vi "抓圓.vi"(0 "Image In":T3, 1 "Process":T8(ring), 2 "Optimized Mode":bool, 3 "Direction":enum16{"Inner to Outer", "Outer to Inner"}(ring), 5 "ROI":T2, 7 "Coordinate System":T1 {"Measurement System"."Axis Reference" items=["Direct", "Indirect"]; "Measurement System"."Angle (deg)" format="%.2f"; "Measurement System"."Origin"."Y" format="%.2f"; "Measurement System"."Origin"."X" format="%.2f"; "Reference System"."Axis Reference" items=["Direct", "Indirect"]; "Reference System"."Angle (deg)" format="%.2f"; "Reference System"."Origin"."Y" format="%.2f"; "Reference System"."Origin"."X" format="%.2f"}, 9 "Gap":i32=10 min=1 max=300, 11 "error In":errorcluster, 12 "Edge Options":T6={"Edge Polarity"=0, "Kernel Size"=3, "Width"=3, "Minimum Edge Strength"=10.0, "Interpolation Type"=enum."Bilinear Fixed", "Data Processing Method"=enum."Average"} {"Edge Polarity" items=["All Edges", "Rising Edges", "Falling Edges"]; "Minimum Edge Strength" format="%.2f"; "Width" step=2; "Kernel Size" step=2}, 13 "Point Diameter (5)":u32=5 min=3 max=1000) -> (4 "Imag e Out":T3, 6 "Line Profile":T4(graph), 10 "Gradient Information":dbl[][](graph), 14 "Ellipse":T5 {"Minor Axis"."Point 2"."Y" format="%.2f"; "Minor Axis"."Point 2"."X" format="%.2f"; "Minor Axis"."Point 1"."Y" format="%.2f"; "Minor Axis"."Point 1"."X" format="%.2f"; "Major Axis"."Point 2"."Y" format="%.2f"; "Major Axis"."Point 2"."X" format="%.2f"; "Major Axis"."Point 1"."Y" format="%.2f"; "Major Axis"."Point 1"."X" format="%.2f"; "Center"."Y" format="%.2f"; "Center"."X" format="%.2f"}, 15 "error out":errorcluster)   [LabVIEW 2015]
uses:
  <vilib>/vision/Measure.llb/Edge Options.ctl
  <vilib>/vision/Measure.llb/Edge Polarity.ctl
  <vilib>/vision/Image Controls.llb/IMAQ Image.ctl
  <vilib>/Analysis/coordinate.llb/2D Cartesian Coordinate Rotation (Scalar).vi
  <vilib>/vision/NI_Vision_Development_Module.lvlib
  <vilib>/Analysis/NI_AALPro.lvlib
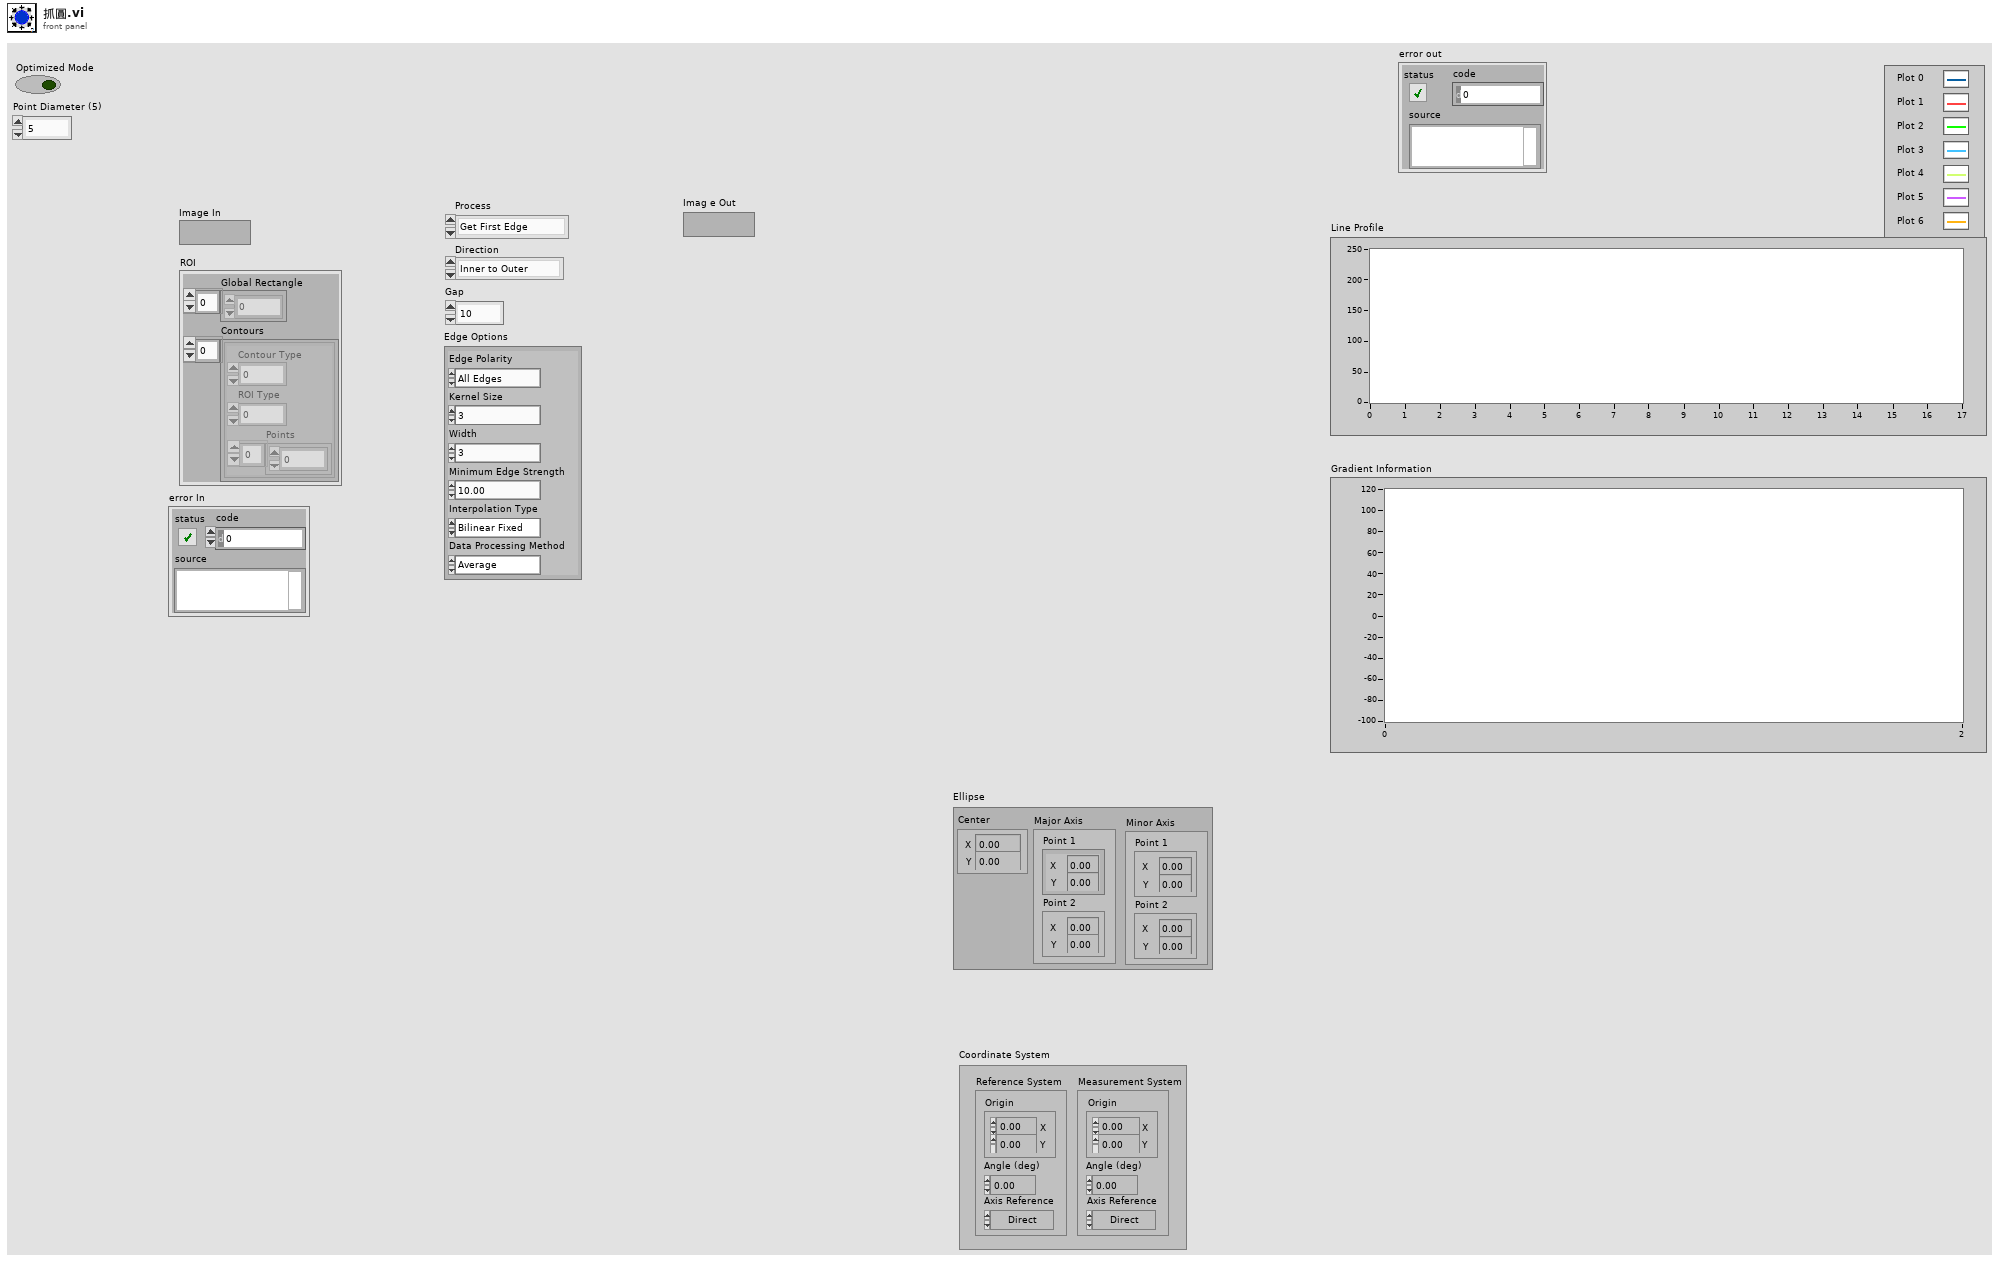
[diagram p1: front panel]
types:
  T1 = typedef "IMAQ Coordinate System" = cluster{"Reference System":cluster{"Origin":cluster{"X":sgl, "Y":sgl}, "Angle (deg)":sgl, "Axis Reference":u32}, "Measurement System":cluster{"Origin":cluster{"X":sgl, "Y":sgl}, "Angle (deg)":sgl, "Axis Reference":u32}}
  T2 = cluster{"Global Rectangle":i32[], "Contours":cluster{"Contour Type":u32, "ROI Type":u32, "Points":i32[]}[]}
  T3 = typedef "IMAQ Image.ctl" = refnum<image>
  T4 = cluster{"x0":sgl, "dx":sgl, "Pixels Line":sgl[]}[]
  T5 = cluster{"Center":cluster{"X":sgl, "Y":sgl}, "Major Axis":cluster{"Point 1":cluster{"X":sgl, "Y":sgl}, "Point 2":cluster{"X":sgl, "Y":sgl}}, "Minor Axis":cluster{"Point 1":cluster{"X":sgl, "Y":sgl}, "Point 2":cluster{"X":sgl, "Y":sgl}}}
  T6 = typedef "Edge Options.ctl" = cluster{"Edge Polarity":T7, "Kernel Size":u32, "Width":u32, "Minimum Edge Strength":sgl, "Interpolation Type":enum32{"Zero Order", "Bilinear", "Quadratic", "Cubic", "Bilinear Fixed"}, "Data Processing Method":enum32{"Average", "Median"}}
  T7 = typedef "Edge Polarity.ctl" = u32
  T8 = enum16{"Get First Edge", "Get First + Last Edge", "Get All Edges", "Get Best Edge"}
  T9 = typedef "IMAQ Point" = cluster{"X":sgl, "Y":sgl}
  T10 = cluster{"Point 1":cluster{"x":dbl, "y":dbl}, "Point 2":cluster{"x":dbl, "y":dbl}}
  T11 = typedef "IMAQ Line" = cluster{"Start X":i32, "Start Y":i32, "End X":i32, "End Y":i32}
  T12 = cluster{"Origin":cluster{"X":sgl, "Y":sgl}, "Angle (deg)":sgl, "Axis Reference":u32}
  T13 = typedef "ROI Descriptor" = cluster{"Global Rectangle":i32[], "Contours":cluster{"ID":enum32{"External", "Internal"}, "Type":u32, "Coordinates":i32[]}[]}
  T14 = typedef "IMAQ Circle" = cluster{"Center X":i32, "Center Y":i32, "Inner Radius":i32, "Outer Radius":i32, "Start Angle":dbl, "End Angle":dbl}
  T15 = typedef "Edge New.ctl" = cluster{"Location (Pixel)":cluster{"X":sgl, "Y":sgl}, "Location (Real-World)":cluster{"X":sgl, "Y":sgl}, "Distance (Pixel)":dbl, "Distance (Real-World)":dbl, "Strength":dbl, "Noise":dbl, "Rising?":bool}
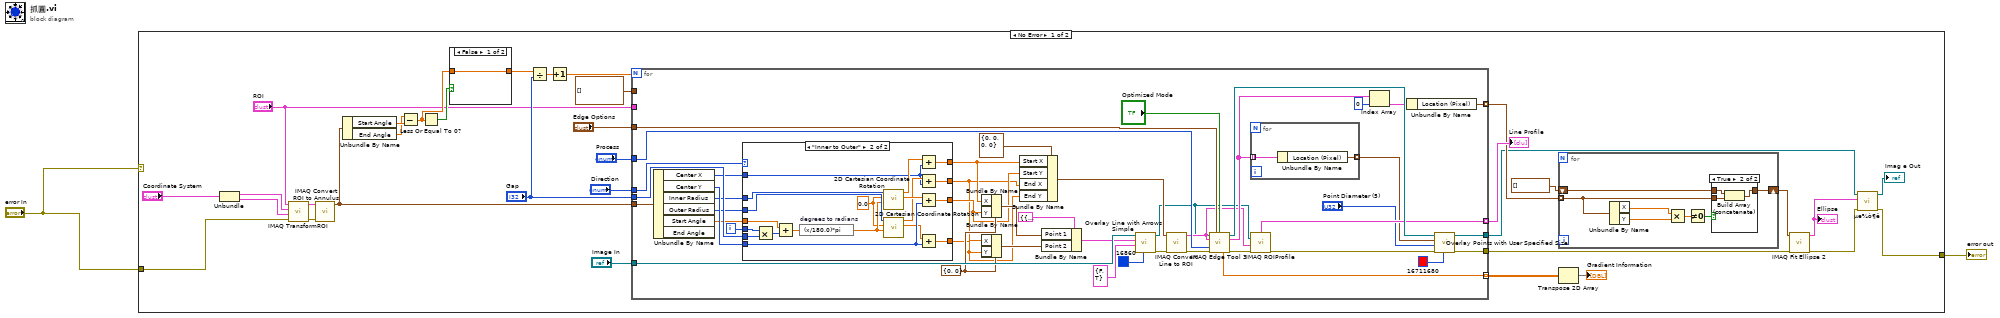
[diagram p0: block diagram]
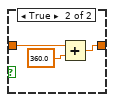
[diagram p2: hidden frame]
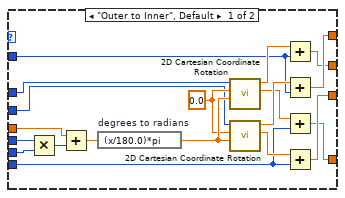
[diagram p4: hidden frame]
diagram:
  n1 = case shown="No Error" "error In" {
    tunnel: "error In" -> [w7 w135]
    tunnel: [w4 w135] -> w2
    frame No Error {
      n2 = Unbundle("Coordinate System") -> ("Reference System"=w13:T12, "Measurement System"=w12:T12)
      n3 = call "IMAQ TransformROI"("error in (no error)"=w7, "New Reference"=w12, "Base Reference"=w13, "ROI Descriptor"="ROI") -> ("error out"=w9:errorcluster, "ROI Descriptor out"=w10:T13)  [unwired: 6 in]
      n4 = call "IMAQ Convert ROI to Annulus"("error in (no error)"=w9, "ROI Descriptor"=w10) -> ("Annulus"=w8:T14)  [unwired: 7 in, 1 out]
      n5 = Unbundle By Name(w8) -> ("Start Angle"=w21:dbl, "End Angle"=w5:dbl)
      n6 = Subtract(x=w5, y=w21) -> (x-y=w15:dbl)
      n7 = Less Or Equal To 0?(x=w15) -> (x <= 0?=w16:bool)
      n8 = case shown="False" w16 {
        tunnel: w15 -> [w36 w38]
        tunnel: [w36 w37] -> w14
        frame False {
        }
        frame True {
          n9 = Add(x=w38, y=360.0) -> (x+y=w37:dbl)
        }
      }
      n10 = Divide(x=w14, y="Gap") -> (x/y=w22:dbl)
      n11 = Increment(x=w22) -> (x+1=w29:dbl)
      n12 = for {
        N: w29 -> [_]
        tunnel: "Direction" -> [w79]
        tunnel: [w89] -> w18
        tunnel: "Image In" -> [w80]
        tunnel: "ROI" -> [_]
        tunnel: [w88] -> w25
        tunnel: "Process" -> [w90]
        tunnel: "Edge Options" -> [w87]
        tunnel: [w86] -> w28 mode=indexing
        tunnel: [w85] -> w30 mode=indexing
        tunnel: [w84] -> w27 mode=indexing
        tunnel: "Gap" -> [w77]
        tunnel: w8 -> [w75]
        tunnel: T9[] [] ("Rectangle Points") -> [_]
        i -> [w76]
        w72 = cluster{"X":i32, "Y":i32} {"X"=0, "Y"=0} ("Start Point")
        n13 = Unbundle By Name(w75) -> ("Center X"=w56:i32, "Center Y"=w55:i32, "Inner Radius"=w54:i32, "Outer Radius"=w53:i32, "Start Angle"=w52:dbl)  [unwired: 1 out]
        n14 = case shown="\"Inner to Outer\"" w79 {
          tunnel: w55 -> [w97 w132]
          tunnel: w54 -> [w96 w131]
          tunnel: w53 -> [w95 w130]
          tunnel: w52 -> [w100 w129]
          tunnel: w77 -> [w98 w128]
          tunnel: w76 -> [w99 w119]
          tunnel: [w105 w114] -> w64
          tunnel: [w103 w118] -> w62
          tunnel: w56 -> [w101 w117]
          tunnel: [w102 w116] -> w61
          tunnel: [w104 w115] -> w63
          frame "Outer to Inner", Default {
            w108 = 0.0 ("y")
            n15 = Multiply(x=w99, y=w98) -> (x*y=w107:i32)
            n16 = Add(x=w100, y=w107) -> (x+y=w106:dbl)
            n17 = expression code="(x/180.0)*pi" "degrees to radians"(w106) -> (w109:dbl)
            n18 = call-poly <vilib>:"2D Cartesian Coordinate Rotation.vi"("theta"=w109, "y"=w108, "x"=w96) -> ("y out"=w111:dbl, "x out"=w110:dbl)  [unwired: 6 in, 1 out]
            n19 = call-poly <vilib>:"2D Cartesian Coordinate Rotation.vi"("theta"=w109, "y"=w108, "x"=w95) -> ("y out"=w112:dbl, "x out"=w113:dbl)  [unwired: 6 in, 1 out]
            n20 = Add(x=w110, y=w101) -> (x+y=w102:dbl)
            n21 = Add(x=w113, y=w101) -> (x+y=w105:dbl)
            n22 = Add(x=w111, y=w97) -> (x+y=w103:dbl)
            n23 = Add(x=w112, y=w97) -> (x+y=w104:dbl)
          }
          frame "Inner to Outer" {
            w122 = 0.0 ("y")
            n24 = Multiply(x=w119, y=w128) -> (x*y=w121:i32)
            n25 = Add(x=w129, y=w121) -> (x+y=w120:dbl)
            n26 = expression code="(x/180.0)*pi" "degrees to radians"(w120) -> (w123:dbl)
            n27 = call-poly <vilib>:"2D Cartesian Coordinate Rotation.vi"("theta"=w123, "y"=w122, "x"=w131) -> ("y out"=w126:dbl, "x out"=w127:dbl)  [unwired: 6 in, 1 out]
            n28 = call-poly <vilib>:"2D Cartesian Coordinate Rotation.vi"("theta"=w123, "y"=w122, "x"=w130) -> ("y out"=w125:dbl, "x out"=w124:dbl)  [unwired: 6 in, 1 out]
            n29 = Add(x=w127, y=w117) -> (x+y=w114:dbl)
            n30 = Add(x=w124, y=w117) -> (x+y=w116:dbl)
            n31 = Add(x=w126, y=w132) -> (x+y=w115:dbl)
            n32 = Add(x=w125, y=w132) -> (x+y=w118:dbl)
          }
        }
        n33 = Bundle By Name(cluster=w72, "X"=w64, "Y"=w63) -> (w70:cluster{"X":i32, "Y":i32})
        n34 = Bundle By Name(cluster=w72, "X"=w61, "Y"=w62) -> (w71:cluster{"X":i32, "Y":i32})
        n35 = Bundle By Name(cluster=T11 {"Start X"=0, "Start Y"=0, "End X"=0, "End Y"=0} ("Line"), "Start X"=w64, "Start Y"=w63, "End X"=w61, "End Y"=w62) -> (w73:T11)
        n36 = Bundle By Name(cluster=T10 {"Point 1"={"x"=50.0, "y"=50.0}, "Point 2"={"x"=70.0, "y"=70.0}} ("Line Coordinates"), "Point 1"=w70, "Point 2"=w71) -> (w67:T10)
        n37 = call "Overlay Line with Arrows Simple.vi"("Color"=u32 16860, "Arrows"=cluster{"Start point":bool, "End point":bool} {"Start point"=FALSE, "End point"=TRUE}, "Line Coordinates"=w67, "Image In"=w80) -> ("error out"=w65:errorcluster, "Image Out"=w66:T3)  [unwired: 6 in]
        n38 = call "IMAQ Convert Line to ROI"("error in (no error)"=w65, "Line"=w73) -> ("error out"=w82:errorcluster, "ROI Descriptor"=w81:T13)  [unwired: 7 in]
        n39 = call "IMAQ Edge Tool 3"("Image"=w66, "Edge Options"=w87, "Optimized Mode"="Optimized Mode", "ROI Descriptor"=w81, "Process"=w90, "error in (no error)"=w82) -> ("Image (duplicate)"=w91:T3, "Edge Information"=w94:T15[], "Gradient Values"=w85:dbl[], "error out"=w83:errorcluster)  [unwired: 5 in, 1 out]
        n40 = for {
          tunnel: w94 -> [w134] mode=indexing
          tunnel: [w133] -> w57 mode=indexing
          n41 = Unbundle By Name(w134) -> ("Location (Pixel)"=w133:cluster{"X":sgl, "Y":sgl})
        }
        n42 = call "IMAQ ROIProfile"("error in (no error)"=w83, "ROI Descriptor"=w81, "Image"=w66) -> ("error out"=w93:errorcluster, "ROI Graph"=w86:cluster{"x0":sgl, "dx":sgl, "Pixels Line":sgl[]})  [unwired: 1 in, 3 out]
        n43 = Index Array(array=w94, index=0) -> (element=w58:T15)
        n44 = Unbundle By Name(w58) -> ("Location (Pixel)"=w84:cluster{"X":sgl, "Y":sgl})
        n45 = call "Overlay Points with User Specified Size.vi"("Color"=u32 16711680, "error in"=w93, "Point Diameter (5)"="Point Diameter (5)", "Points"=w57, "Image In"=w91) -> ("error out"=w88:errorcluster, "Image Out"=w89:T3)  [unwired: 5 in]
      }
      "Line Profile" <- w28
      n46 = for {
        tunnel: w27 -> [w42] mode=indexing
        shift-right: [w41] -> w26
        shift-left: cluster{"X":sgl, "Y":sgl}[] [] -> [w40]
        n47 = Unbundle By Name(w42) -> ("X"=w46:sgl, "Y"=w45:sgl)
        n48 = Multiply(x=w46, y=w45) -> (x*y=w44:sgl)
        n49 = Not Equal To 0?(x=w44) -> (x != 0?=w43:bool)
        n50 = case shown="True" w43 {
          tunnel: w42 -> [_ w50]
          tunnel: [w47 w49] -> w41
          tunnel: w40 -> [w47 w48]
          frame False {
          }
          frame True {
            n51 = Build Array (concatenate)(w48, w50) -> (w49:cluster{"X":sgl, "Y":sgl}[])
          }
        }
      }
      n52 = Transpose 2D Array(2D array=w30) -> (transposed array=→"Gradient Information":dbl[][])
      n53 = call "IMAQ Fit Ellipse 2"("error in (no error)"=w25, "Radial Points"=w26) -> ("error out"=w3:errorcluster, "Ellipse"=w19:T5)  [unwired: 4 in, 4 out]
      "Ellipse" <- w19
      n54 = call "µe¾ò¶ê.vi"("error in (no error)"=w3, "Ellipse"=w19, "Image In"=w18) -> ("error out"=w4:errorcluster, "Image"=→"Imag e Out":T3)  [unwired: 7 in]
    }
    frame Error {
    }
  }
  "error out" <- w2
